vi "LED_quickCompare.vi"() -> ()   [LabVIEW 2012]
panel:
  in  "Device Area 2 (m2)":dbl=3e-06
  out "current efficiency (Cd/A) 2":dbl[](array[numeric])
  out "current density (mA/cm2) 2":dbl[](array[numeric])
  out "uW 2":dbl[](array[numeric])
  out "luminance (Cd/m2) 2":dbl[](array[numeric])
  out "candela (Cd) 2":dbl[](array[numeric])
  out "array 2":dbl[][](array[numeric])
  out "substring 2":string
  out "current 2":dbl[](array[numeric])=[6.47737e-06, 2.6904e-06, 1.39949e-05, 2.68063e-06, 9.1124e-06, 1.90109e-14, 1.97383e-05, 3.27886e-05, 1.52434e-14, 1.39406e-14, 1.38211e-06, 5.60771e-06, 1.05119e-14, 5.17343e-06, 8.75954e-15, 7.94526e-06, 3.52097e-06, 6.93229e-15, 6.13103e-06, 2.17143e-06, 5.79229e-15, 4.74349e-06, 1.31046e-05, 1.46246e-05, 1.64051e-05, 7.16029e-06, 1.45269e-05, 1.8848e-05, 1.69046e-05, 2.94011e-05, 3.6784e-05, 4.04863e-05, 4.8336e-05, 7.44474e-05, 8.9224e-05, 0.00011096, 0.000158297, 0.000223114, 0.000309646, 0.000425274, 0.00055936, 0.00072124, 0.000872154, 0.00098648, 0.00107, 0.00113, 0.00114, 0.00113, 0.00111, 0.00107, 0.00102, 0.000982897, 0.000954886, 0.00092416, 0.000901903, 0.000883446, 0.000877257, 0.000876606, 0.000867594, 0.00086716, 0.00086032, 0.000838063, 0.000814503, 0.000782583, 0.000746537, 0.000713966, 0.000685194, 0.000641549, 0.00060116, 0.000566634, 0.00053808, 0.00051224, 0.000480646, 0.000459474, 0.000436566, 0.000413983, 0.000402691, 0.000382714, 0.0003648, 0.000347754, 0.000340697, 0.000318657, 0.000305303, 0.000288366, 0.000271103, 0.000258183, 0.000245046, 0.000230497, 0.00021584, 0.000209109, 0.000197383, 0.000185223, 0.000174909, 0.000168069, 0.000157211, 0.000145051, 0.00014288, 0.000137777, 0.000130069, 0.000120731, 0.000116931, 0.00011324, 0.000107421, 9.73017e-05, 9.4924e-05, 8.8844e-05, 8.98971e-05, 8.97126e-05, 7.89206e-05, 7.94309e-05, 7.32097e-05, 6.66629e-05, 6.16903e-05, 5.57949e-05, 6.20811e-05, 5.63594e-05, 5.13543e-05, 4.87377e-05, 4.47097e-05, 4.64794e-05, 4.35371e-05, 4.20389e-05, 4.2408e-05, 3.41891e-05, 3.3744e-05, 3.43086e-05, 3.08126e-05, 3.16377e-05, 3.192e-05, 3.3744e-05, 2.9792e-05, 2.53949e-05, 2.44829e-05, 2.15949e-05, 1.91954e-05, 2.39617e-05, 2.4244e-05, 2.0216e-05, 1.47983e-05, 1.92823e-05, 1.94777e-05, 1.04098e-05, 1.98794e-05, 1.80771e-05, 1.34303e-05, 1.30177e-05, 1.81314e-05, 1.28549e-05, 1.38971e-05, 1.89891e-05, 1.748e-05, 1.85766e-05, 1.28983e-05, 8.3524e-06, 7.15051e-06, 6.38943e-06, 1.80337e-05, 1.7784e-05, 8.00931e-06, 1.04055e-05, 1.15629e-05, 3.42869e-06, 7.79109e-06, 1.20514e-05, 6.23526e-06, 5.57297e-06, 1.03979e-05, 9.60097e-06, 3.77611e-06, 4.99971e-06, 1.86091e-05, 7.97783e-06, 4.75326e-06, 1.34954e-05, 4.08663e-06, 5.80206e-06, 8.21669e-06, 3.33531e-06, 5.61531e-06, 6.92903e-06, 6.47954e-06, 5.80206e-06, 3.11817e-06, 7.95177e-06, 1.47983e-05, 1.30177e-05, 4.10617e-06, 1.09766e-06, 1.23337e-14, 4.39606e-06, 2.204e-06, 3.85646e-06, 1.12371e-05, 2.84674e-06, 1.52e-14, 1.57537e-14, 1.62097e-14, 1.67526e-05, 1.65789e-14, 3.78263e-06, 6.14189e-06]
  out "voltage 2":dbl[](array[numeric])=[380.0, 382.0, 384.0, 386.0, 388.0, 390.0, 392.0, 394.0, 396.0, 398.0, 400.0, 402.0, 404.0, 406.0, 408.0, 410.0, 412.0, 414.0, 416.0, 418.0, 420.0, 422.0, 424.0, 426.0, 428.0, 430.0, 432.0, 434.0, 436.0, 438.0, 440.0, 442.0, 444.0, 446.0, 448.0, 450.0, 452.0, 454.0, 456.0, 458.0, 460.0, 462.0, 464.0, 466.0, 468.0, 470.0, 472.0, 474.0, 476.0, 478.0, 480.0, 482.0, 484.0, 486.0, 488.0, 490.0, 492.0, 494.0, 496.0, 498.0, 500.0, 502.0, 504.0, 506.0, 508.0, 510.0, 512.0, 514.0, 516.0, 518.0, 520.0, 522.0, 524.0, 526.0, 528.0, 530.0, 532.0, 534.0, 536.0, 538.0, 540.0, 542.0, 544.0, 546.0, 548.0, 550.0, 552.0, 554.0, 556.0, 558.0, 560.0, 562.0, 564.0, 566.0, 568.0, 570.0, 572.0, 574.0, 576.0, 578.0, 580.0, 582.0, 584.0, 586.0, 588.0, 590.0, 592.0, 594.0, 596.0, 598.0, 600.0, 602.0, 604.0, 606.0, 608.0, 610.0, 612.0, 614.0, 616.0, 618.0, 620.0, 622.0, 624.0, 626.0, 628.0, 630.0, 632.0, 634.0, 636.0, 638.0, 640.0, 642.0, 644.0, 646.0, 648.0, 650.0, 652.0, 654.0, 656.0, 658.0, 660.0, 662.0, 664.0, 666.0, 668.0, 670.0, 672.0, 674.0, 676.0, 678.0, 680.0, 682.0, 684.0, 686.0, 688.0, 690.0, 692.0, 694.0, 696.0, 698.0, 700.0, 702.0, 704.0, 706.0, 708.0, 710.0, 712.0, 714.0, 716.0, 718.0, 720.0, 722.0, 724.0, 726.0, 728.0, 730.0, 732.0, 734.0, 736.0, 738.0, 740.0, 742.0, 744.0, 746.0, 748.0, 750.0, 752.0, 754.0, 756.0, 758.0, 760.0, 762.0, 764.0, 766.0, 768.0, 770.0, 772.0, 774.0, 776.0, 778.0, 780.0]
  in  "file 2":path
  out "Current Efficiency vs Luminance/Current Density":cluster{"Y":dbl[], "Y":dbl[]}[](graph)
  out "Current Density/Luminance vs Voltage":cluster{"Y":dbl[], "Y":dbl[]}[](graph)
  out "current efficiency (Cd/A)":dbl[](array[numeric])
  out "current density (mA/cm2)":dbl[](array[numeric])
  in  "Device Area 1 (m2)":dbl=3e-06
  out "uW":dbl[](array[numeric])
  out "luminance (Cd/m2)":dbl[](array[numeric])
  out "candela (Cd)":dbl[](array[numeric])
  out "array":dbl[][](array[numeric])
  out "substring":string
  out "current":dbl[](array[numeric])=[6.47737e-06, 2.6904e-06, 1.39949e-05, 2.68063e-06, 9.1124e-06, 1.90109e-14, 1.97383e-05, 3.27886e-05, 1.52434e-14, 1.39406e-14, 1.38211e-06, 5.60771e-06, 1.05119e-14, 5.17343e-06, 8.75954e-15, 7.94526e-06, 3.52097e-06, 6.93229e-15, 6.13103e-06, 2.17143e-06, 5.79229e-15, 4.74349e-06, 1.31046e-05, 1.46246e-05, 1.64051e-05, 7.16029e-06, 1.45269e-05, 1.8848e-05, 1.69046e-05, 2.94011e-05, 3.6784e-05, 4.04863e-05, 4.8336e-05, 7.44474e-05, 8.9224e-05, 0.00011096, 0.000158297, 0.000223114, 0.000309646, 0.000425274, 0.00055936, 0.00072124, 0.000872154, 0.00098648, 0.00107, 0.00113, 0.00114, 0.00113, 0.00111, 0.00107, 0.00102, 0.000982897, 0.000954886, 0.00092416, 0.000901903, 0.000883446, 0.000877257, 0.000876606, 0.000867594, 0.00086716, 0.00086032, 0.000838063, 0.000814503, 0.000782583, 0.000746537, 0.000713966, 0.000685194, 0.000641549, 0.00060116, 0.000566634, 0.00053808, 0.00051224, 0.000480646, 0.000459474, 0.000436566, 0.000413983, 0.000402691, 0.000382714, 0.0003648, 0.000347754, 0.000340697, 0.000318657, 0.000305303, 0.000288366, 0.000271103, 0.000258183, 0.000245046, 0.000230497, 0.00021584, 0.000209109, 0.000197383, 0.000185223, 0.000174909, 0.000168069, 0.000157211, 0.000145051, 0.00014288, 0.000137777, 0.000130069, 0.000120731, 0.000116931, 0.00011324, 0.000107421, 9.73017e-05, 9.4924e-05, 8.8844e-05, 8.98971e-05, 8.97126e-05, 7.89206e-05, 7.94309e-05, 7.32097e-05, 6.66629e-05, 6.16903e-05, 5.57949e-05, 6.20811e-05, 5.63594e-05, 5.13543e-05, 4.87377e-05, 4.47097e-05, 4.64794e-05, 4.35371e-05, 4.20389e-05, 4.2408e-05, 3.41891e-05, 3.3744e-05, 3.43086e-05, 3.08126e-05, 3.16377e-05, 3.192e-05, 3.3744e-05, 2.9792e-05, 2.53949e-05, 2.44829e-05, 2.15949e-05, 1.91954e-05, 2.39617e-05, 2.4244e-05, 2.0216e-05, 1.47983e-05, 1.92823e-05, 1.94777e-05, 1.04098e-05, 1.98794e-05, 1.80771e-05, 1.34303e-05, 1.30177e-05, 1.81314e-05, 1.28549e-05, 1.38971e-05, 1.89891e-05, 1.748e-05, 1.85766e-05, 1.28983e-05, 8.3524e-06, 7.15051e-06, 6.38943e-06, 1.80337e-05, 1.7784e-05, 8.00931e-06, 1.04055e-05, 1.15629e-05, 3.42869e-06, 7.79109e-06, 1.20514e-05, 6.23526e-06, 5.57297e-06, 1.03979e-05, 9.60097e-06, 3.77611e-06, 4.99971e-06, 1.86091e-05, 7.97783e-06, 4.75326e-06, 1.34954e-05, 4.08663e-06, 5.80206e-06, 8.21669e-06, 3.33531e-06, 5.61531e-06, 6.92903e-06, 6.47954e-06, 5.80206e-06, 3.11817e-06, 7.95177e-06, 1.47983e-05, 1.30177e-05, 4.10617e-06, 1.09766e-06, 1.23337e-14, 4.39606e-06, 2.204e-06, 3.85646e-06, 1.12371e-05, 2.84674e-06, 1.52e-14, 1.57537e-14, 1.62097e-14, 1.67526e-05, 1.65789e-14, 3.78263e-06, 6.14189e-06]
  out "voltage":dbl[](array[numeric])=[380.0, 382.0, 384.0, 386.0, 388.0, 390.0, 392.0, 394.0, 396.0, 398.0, 400.0, 402.0, 404.0, 406.0, 408.0, 410.0, 412.0, 414.0, 416.0, 418.0, 420.0, 422.0, 424.0, 426.0, 428.0, 430.0, 432.0, 434.0, 436.0, 438.0, 440.0, 442.0, 444.0, 446.0, 448.0, 450.0, 452.0, 454.0, 456.0, 458.0, 460.0, 462.0, 464.0, 466.0, 468.0, 470.0, 472.0, 474.0, 476.0, 478.0, 480.0, 482.0, 484.0, 486.0, 488.0, 490.0, 492.0, 494.0, 496.0, 498.0, 500.0, 502.0, 504.0, 506.0, 508.0, 510.0, 512.0, 514.0, 516.0, 518.0, 520.0, 522.0, 524.0, 526.0, 528.0, 530.0, 532.0, 534.0, 536.0, 538.0, 540.0, 542.0, 544.0, 546.0, 548.0, 550.0, 552.0, 554.0, 556.0, 558.0, 560.0, 562.0, 564.0, 566.0, 568.0, 570.0, 572.0, 574.0, 576.0, 578.0, 580.0, 582.0, 584.0, 586.0, 588.0, 590.0, 592.0, 594.0, 596.0, 598.0, 600.0, 602.0, 604.0, 606.0, 608.0, 610.0, 612.0, 614.0, 616.0, 618.0, 620.0, 622.0, 624.0, 626.0, 628.0, 630.0, 632.0, 634.0, 636.0, 638.0, 640.0, 642.0, 644.0, 646.0, 648.0, 650.0, 652.0, 654.0, 656.0, 658.0, 660.0, 662.0, 664.0, 666.0, 668.0, 670.0, 672.0, 674.0, 676.0, 678.0, 680.0, 682.0, 684.0, 686.0, 688.0, 690.0, 692.0, 694.0, 696.0, 698.0, 700.0, 702.0, 704.0, 706.0, 708.0, 710.0, 712.0, 714.0, 716.0, 718.0, 720.0, 722.0, 724.0, 726.0, 728.0, 730.0, 732.0, 734.0, 736.0, 738.0, 740.0, 742.0, 744.0, 746.0, 748.0, 750.0, 752.0, 754.0, 756.0, 758.0, 760.0, 762.0, 764.0, 766.0, 768.0, 770.0, 772.0, 774.0, 776.0, 778.0, 780.0]
  in  "file 1":path
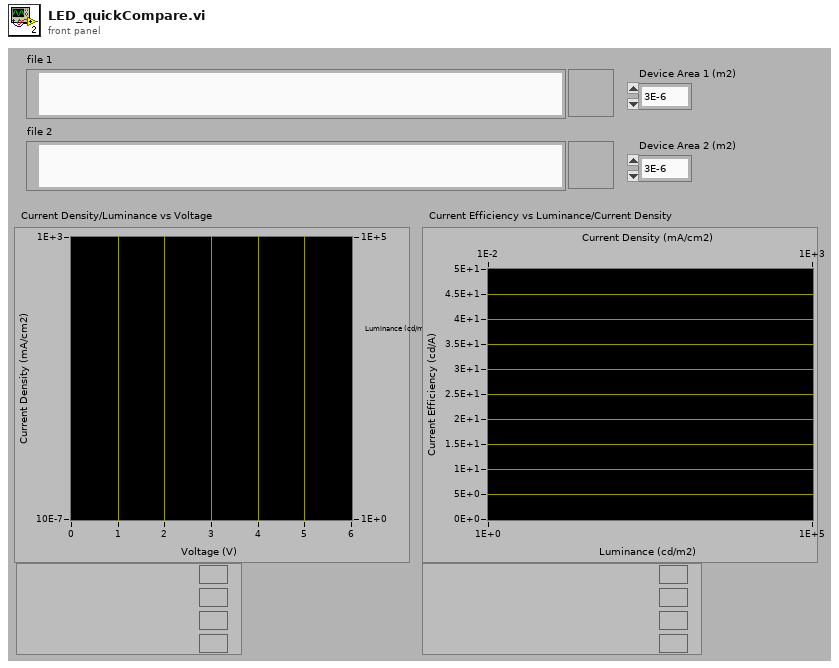
[diagram p1: front panel]
types:
  T1 = cluster{"luminance (Cd/m2)":dbl[], "current efficiency (Cd/A)":dbl[]}
  T2 = cluster{"current density (mA/cm2)":dbl[], "current efficiency (Cd/A)":dbl[]}
  T3 = cluster{"luminance (Cd/m2) 2":dbl[], "current efficiency (Cd/A) 2":dbl[]}
  T4 = cluster{"current density (mA/cm2) 2":dbl[], "current efficiency (Cd/A) 2":dbl[]}
  T5 = cluster{"current density (mA/cm2) 2":dbl[], "current efficiency (Cd/A) 2":dbl[]}[]
  T6 = cluster{"voltage":dbl[], "luminance (Cd/m2)":dbl[]}
  T7 = cluster{"voltage 2":dbl[], "luminance (Cd/m2) 2":dbl[]}
  T8 = cluster{"voltage 2":dbl[], "luminance (Cd/m2) 2":dbl[]}[]
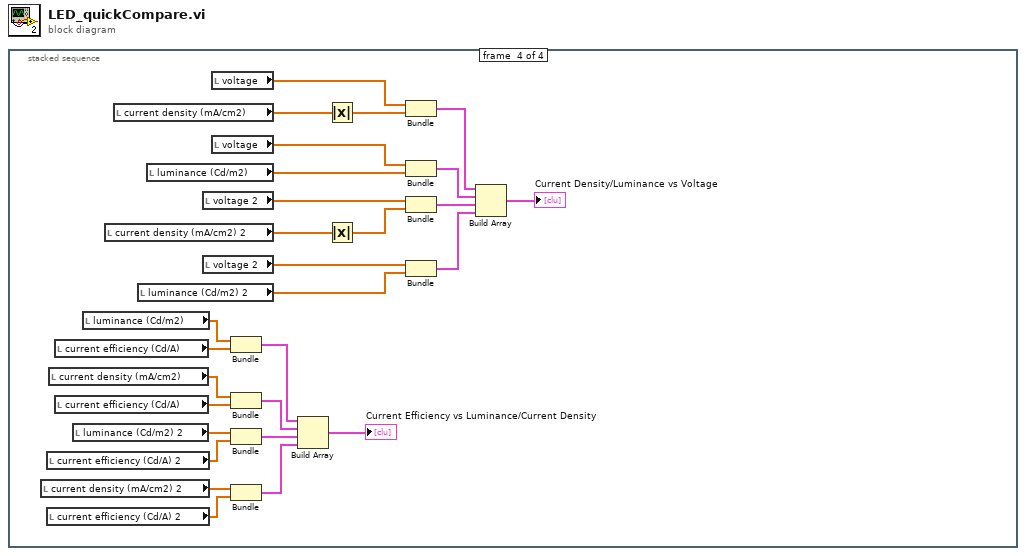
[diagram p0: block diagram]
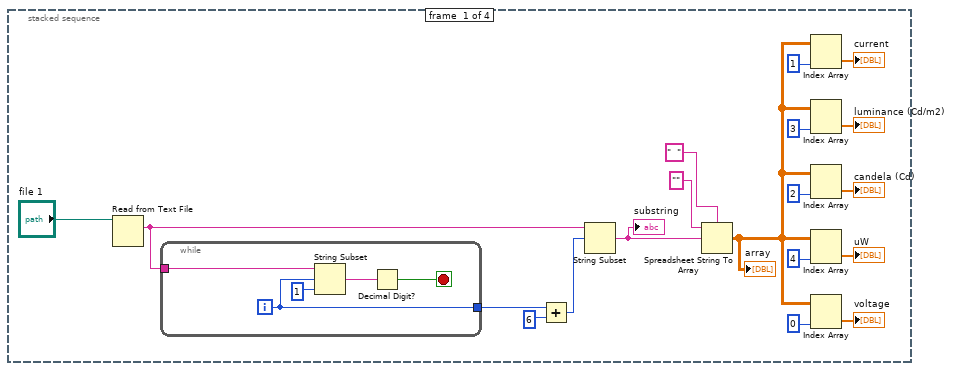
[diagram p2: hidden frame]
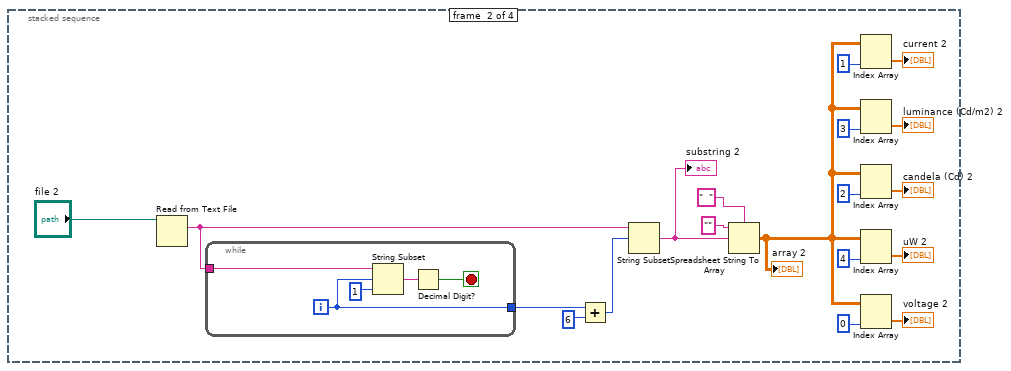
[diagram p3: hidden frame]
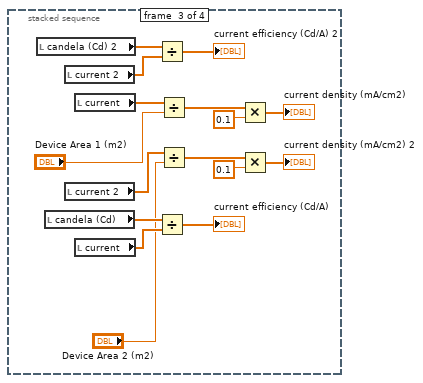
[diagram p4: hidden frame]
diagram:
  n1 = stacked-sequence {
    frame #0 {
      n2 = Read from Text File(file (use dialog)="file 1") -> (text=w15:string)  [unwired: 3 in, 3 out]
      n3 = while {
        tunnel: w15 -> [w24]
        tunnel: [w20] -> w12
        i -> [w20]
        stop <- w21 stop-if-true
        n4 = String Subset(string=w24, offset (0)=w20, length (rest)=1 ("length (rest)")) -> (substring=w22:string)
        n5 = Decimal Digit?(1:w22) -> (0:w21:bool)
      }
      n6 = Add(x=w12, y=6) -> (x+y=w10:i32)
      n7 = String Subset(string=w15, offset (0)=w10) -> (substring=w13:string)  [unwired: 1 in]
      "substring" <- w13
      n8 = Spreadsheet String To Array(delimiter (Tab)="  ", format string="", spreadsheet string=w13) -> (array=w1:dbl[][])  [unwired: 1 in]
      "array" <- w1
      n9 = Index Array(array=w1, index (col)=1 ("disabled index (col)")) -> (element=→"current":dbl[])  [unwired: 1 in]
      n10 = Index Array(array=w1, index (col)=3 ("disabled index (col)")) -> (element=→"luminance (Cd/m2)":dbl[])  [unwired: 1 in]
      n11 = Index Array(array=w1, index (col)=2 ("disabled index (col)")) -> (element=→"candela (Cd)":dbl[])  [unwired: 1 in]
      n12 = Index Array(array=w1, index (col)=4 ("disabled index (col)")) -> (element=→"uW":dbl[])  [unwired: 1 in]
      n13 = Index Array(array=w1, index (col)=0 ("disabled index (col)")) -> (element=→"voltage":dbl[])  [unwired: 1 in]
    }
    frame #1 {
      n14 = Read from Text File(file (use dialog)="file 2") -> (text=w39:string)  [unwired: 3 in, 3 out]
      n15 = while {
        tunnel: w39 -> [w48]
        tunnel: [w44] -> w36
        i -> [w44]
        stop <- w45 stop-if-true
        n16 = String Subset(string=w48, offset (0)=w44, length (rest)=1 ("length (rest)")) -> (substring=w46:string)
        n17 = Decimal Digit?(1:w46) -> (0:w45:bool)
      }
      n18 = Add(x=w36, y=6) -> (x+y=w34:i32)
      n19 = String Subset(string=w39, offset (0)=w34) -> (substring=w37:string)  [unwired: 1 in]
      "substring 2" <- w37
      n20 = Spreadsheet String To Array(delimiter (Tab)="  ", format string="", spreadsheet string=w37) -> (array=w25:dbl[][])  [unwired: 1 in]
      "array 2" <- w25
      n21 = Index Array(array=w25, index (col)=1 ("disabled index (col)")) -> (element=→"current 2":dbl[])  [unwired: 1 in]
      n22 = Index Array(array=w25, index (col)=3 ("disabled index (col)")) -> (element=→"luminance (Cd/m2) 2":dbl[])  [unwired: 1 in]
      n23 = Index Array(array=w25, index (col)=2 ("disabled index (col)")) -> (element=→"candela (Cd) 2":dbl[])  [unwired: 1 in]
      n24 = Index Array(array=w25, index (col)=4 ("disabled index (col)")) -> (element=→"uW 2":dbl[])  [unwired: 1 in]
      n25 = Index Array(array=w25, index (col)=0 ("disabled index (col)")) -> (element=→"voltage 2":dbl[])  [unwired: 1 in]
    }
    frame #2 {
      n26 = local read "candela (Cd) 2"() -> (w53:dbl[])
      n27 = local read "candela (Cd)"() -> (w60:dbl[])
      n28 = local read "current 2"() -> (w54:dbl[])
      n29 = local read "current 2"() -> (w51:dbl[])
      n30 = local read "current"() -> (w58:dbl[])
      n31 = local read "current"() -> (w61:dbl[])
      n32 = Divide(x=w53, y=w54) -> (x/y=→"current efficiency (Cd/A) 2":dbl[])
      n33 = Divide(x=w60, y=w61) -> (x/y=→"current efficiency (Cd/A)":dbl[])
      n34 = Divide(x=w58, y="Device Area 1 (m2)") -> (x/y=w63:dbl[])
      n35 = Divide(x=w51, y="Device Area 2 (m2)") -> (x/y=w56:dbl[])
      n36 = Multiply(x=w63, y=0.1) -> (x*y=→"current density (mA/cm2)":dbl[])
      n37 = Multiply(x=w56, y=0.1) -> (x*y=→"current density (mA/cm2) 2":dbl[])
    }
    frame #3 {
      n38 = local read "current density (mA/cm2) 2"() -> (w70:dbl[])
      n39 = local read "current efficiency (Cd/A) 2"() -> (w69:dbl[])
      n40 = local read "current efficiency (Cd/A) 2"() -> (w78:dbl[])
      n41 = local read "current density (mA/cm2)"() -> (w67:dbl[])
      n42 = local read "current efficiency (Cd/A)"() -> (w66:dbl[])
      n43 = local read "current efficiency (Cd/A)"() -> (w87:dbl[])
      n44 = local read "luminance (Cd/m2) 2"() -> (w77:dbl[])
      n45 = local read "luminance (Cd/m2)"() -> (w82:dbl[])
      n46 = local read "current density (mA/cm2) 2"() -> (w79:dbl[])
      n47 = local read "current density (mA/cm2)"() -> (w88:dbl[])
      n48 = local read "luminance (Cd/m2) 2"() -> (w72:dbl[])
      n49 = local read "luminance (Cd/m2)"() -> (w68:dbl[])
      n50 = local read "voltage 2"() -> (w71:dbl[])
      n51 = local read "voltage 2"() -> (w80:dbl[])
      n52 = local read "voltage"() -> (w65:dbl[])
      n53 = local read "voltage"() -> (w91:dbl[])
      n54 = Bundle("luminance (Cd/m2)"=w82, "current efficiency (Cd/A)"=w66) -> (w83:T1)  [unwired: 1 in]
      n55 = Bundle("current density (mA/cm2)"=w67, "current efficiency (Cd/A)"=w87) -> (w84:T2)  [unwired: 1 in]
      n56 = Bundle("luminance (Cd/m2) 2"=w77, "current efficiency (Cd/A) 2"=w69) -> (w76:T3)  [unwired: 1 in]
      n57 = Bundle("current density (mA/cm2) 2"=w70, "current efficiency (Cd/A) 2"=w78) -> (w75:T4)  [unwired: 1 in]
      n58 = Build Array(w83, w84, w76, w75) -> (→"Current Efficiency vs Luminance/Current Density":T5)
      n59 = Absolute Value(x=w88) -> (abs(x)=w92:dbl[])
      n60 = Absolute Value(x=w79) -> (abs(x)=w81:dbl[])
      n61 = Bundle("voltage"=w65, w92) -> (w89:cluster{"voltage":dbl[], dbl[]})  [unwired: 1 in]
      n62 = Bundle("voltage"=w91, "luminance (Cd/m2)"=w68) -> (w90:T6)  [unwired: 1 in]
      n63 = Bundle("voltage 2"=w71, w81) -> (w74:cluster{"voltage 2":dbl[], dbl[]})  [unwired: 1 in]
      n64 = Bundle("voltage 2"=w80, "luminance (Cd/m2) 2"=w72) -> (w73:T7)  [unwired: 1 in]
      n65 = Build Array(w89, w90, w74, w73) -> (→"Current Density/Luminance vs Voltage":T8)
    }
  }
